vi "Quadratic interpolation method.vi"(10 "FFT array":dbl[](array[numeric])) -> (2 "Index Bin":dbl)   [LabVIEW 2014]
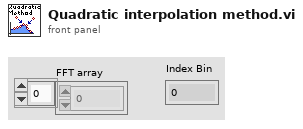
[diagram p1: front panel]
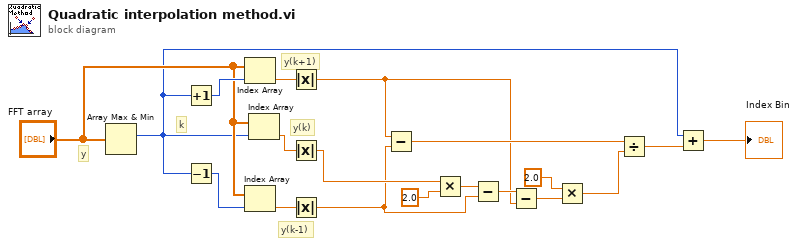
[diagram p0: block diagram]
diagram:
  # "y(k-1)"
  # "y(k+1)"
  # "y(k)"
  # "y"
  # "k"
  n1 = Array Max & Min(array="FFT array") -> (max index (indices)=w1:i32)  [unwired: 3 out]
  n2 = Increment(x=w1) -> (x+1=w19:i32)
  n3 = Decrement(x=w1) -> (x-1=w17:i32)
  n4 = Index Array(array="FFT array", index=w19) -> (element=w15:dbl)
  n5 = Index Array(array="FFT array", index=w17) -> (element=w16:dbl)
  n6 = Index Array(array="FFT array", index=w1) -> (element=w14:dbl)
  n7 = Absolute Value(x=w15) -> (abs(x)=w7:dbl)
  n8 = Absolute Value(x=w14) -> (abs(x)=w12:dbl)
  n9 = Absolute Value(x=w16) -> (abs(x)=w9:dbl)
  n10 = Subtract(x=w7, y=w9) -> (x-y=w13:dbl)
  n11 = Multiply(x=w12, y=2.0) -> (x*y=w10:dbl)
  n12 = Subtract(x=w10, y=w9) -> (x-y=w8:dbl)
  n13 = Subtract(x=w8, y=w7) -> (x-y=w6:dbl)
  n14 = Multiply(x=2.0, y=w6) -> (x*y=w4:dbl)
  n15 = Divide(x=w13, y=w4) -> (x/y=w3:dbl)
  n16 = Add(x=w1, y=w3) -> (x+y=→"Index Bin":dbl)
